vi "Read Data.vi"(8 "error in (no error)":errorcluster, 11 "LakeShore 335 in":refnum<class "LakeShore 335.lvclass">) -> (0 "error out":errorcluster, 2 "Data":waveform(dbl)[](array[waveform]), 3 "LakeShore 335 out":refnum<class "LakeShore 335.lvclass">)   [LabVIEW 2015, in "LakeShore 335.lvclass"]
uses:
  LakeShore 335.lvclass
  LakeShore335 Front Panel Data.ctl
  LakeShore335 Heater Ranges.ctl
  Neocera/Neocera Set Point Aproach.ctl
  OO Devices/Device/Read Controls Snapshot.vi
  Instrument/Read VISA Resource.vi
  OO Devices/Device/Read Control Panel Loaded.vi
  Instrument/Write VISA Resource.vi
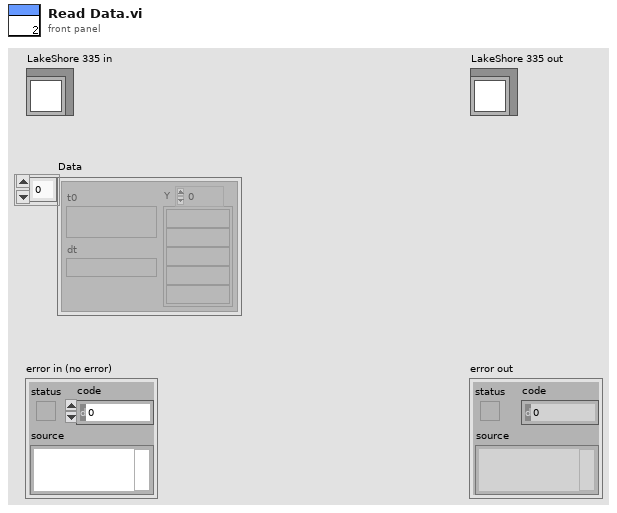
[diagram p1: front panel]
types:
  T1 = typedef "LakeShore335 Front Panel Data.ctl" = cluster{"Heater":bool, "A":bool, "B":bool, " RAW":bool, "Set point":dbl, "Set Heater Range":T2, "Approach":T3, "Ramp rate, K/min":dbl}
  T2 = typedef "LakeShore335 Heater Ranges.ctl" = enum16{"0 (Off)", "1 Low", "2 Medium", "3 High"}
  T3 = typedef "Neocera Set Point Aproach.ctl" = enum16{"Instant", "Ramp"}
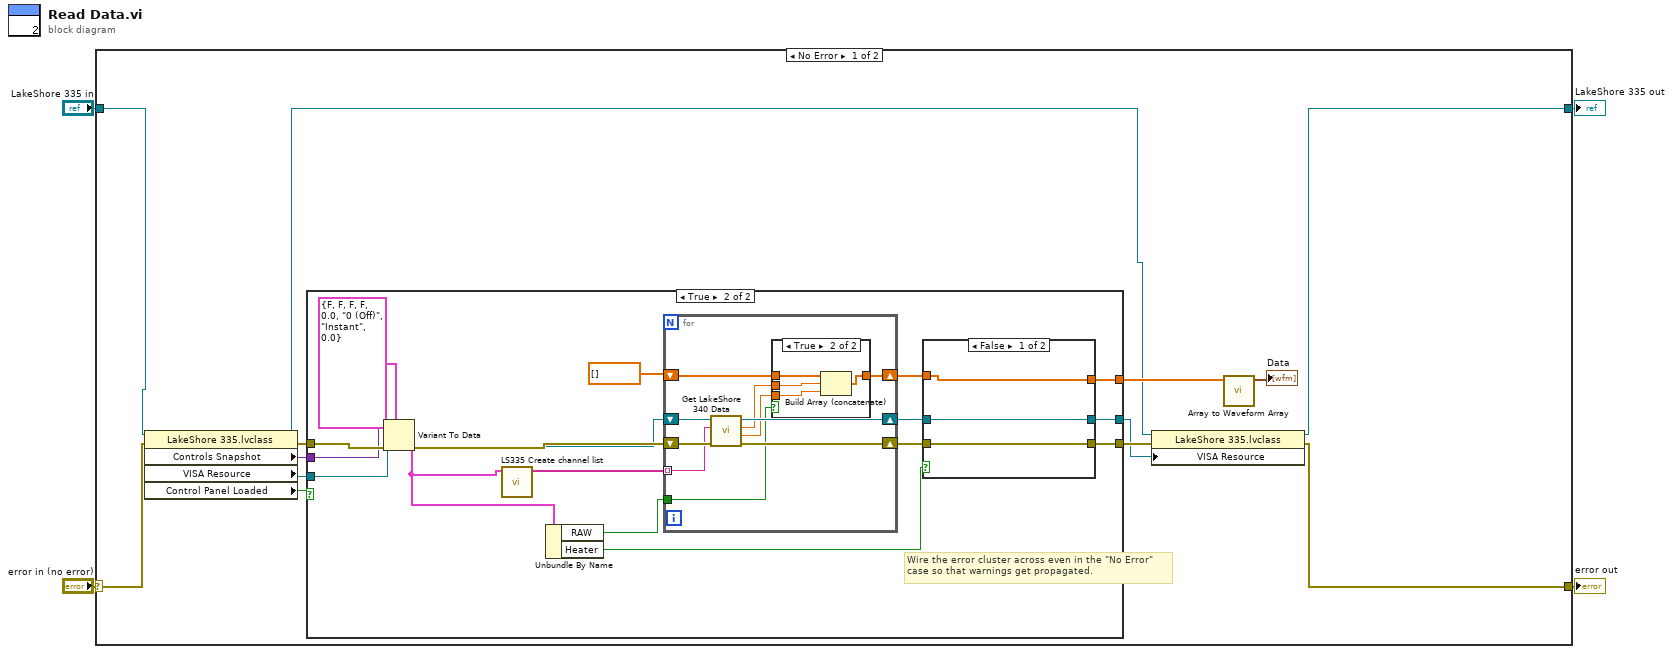
[diagram p0: block diagram]
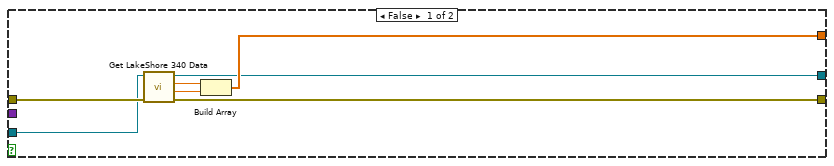
[diagram p2: hidden frame]
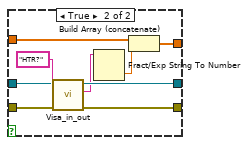
[diagram p3: hidden frame]
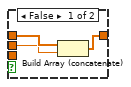
[diagram p4: hidden frame]
diagram:
  n1 = case shown="No Error" "error in (no error)" {
    selector: "error in (no error)" -> [w9 w71]
    tunnel: [w5 w71] -> w3
    tunnel: [w6 w70] -> w1
    tunnel: "LakeShore 335 in" -> [w8 w70]
    frame No Error {
      # "Wire the error cluster across even in the \"No Error\"\ncase so that warnings get propagated."
      n2 = property class="LakeShore 335.lvclass"(reference=w8, error in=w9) -> (reference out=w7:refnum<class "LakeShore 335.lvclass">, error out=w16:errorcluster, "Controls Snapshot"=w15:variant, "VISA Resource"=w12:refnum<visa-resource-name>, "Control Panel Loaded"=w11:bool)
      n3 = case shown="True" w11 {
        tunnel: w16 -> [w24 w40]
        tunnel: w15 -> [_ w39]
        tunnel: [w22 w33] -> w14
        tunnel: [w19 w30] -> w13
        tunnel: w12 -> [w23 w28]
        tunnel: [w18 w27] -> w10
        frame False {
          n4 = call "Get LakeShore 340 Data.vi"("error in (no error)"=w24, "VISA Resource Name"=w23) -> ("error out"=w22:errorcluster, "Raw"=w20:dbl, "Temperature"=w21:dbl, "VISA Resource Name Out"=w18:refnum<visa-resource-name>)  [unwired: 1 in, 5 out]
          n5 = Build Array(w21, w20) -> (w19:dbl[])
        }
        frame True {
          n6 = Variant To Data(error in=w40, type=T1 {"Heater"=FALSE, "A"=FALSE, "B"=FALSE, " RAW"=FALSE, "Set point"=0.0, "Set Heater Range"=enum."0 (Off)", "Approach"=enum."Instant", "Ramp rate, K/min"=0.0} ("Data"), Variant=w39) -> (data=w26:T1, error out=w29:errorcluster)
          n7 = call "LS335 Create channel list.vi"("Data"=w26) -> ("Array"=w25:string[])  [unwired: 10 in]
          n8 = Unbundle By Name(w26) -> ("RAW"=w36:bool, "Heater"=w35:bool)
          n9 = for {
            shift-right: [w62] -> w34
            shift-left: w29 -> [w61]
            shift-right: [w60] -> w32
            shift-left: w28 -> [w59]
            shift-right: [w56] -> w31
            shift-left: dbl[] [] -> [w58]
            tunnel: w36 -> [w54]
            tunnel: w25 -> [w53] mode=indexing
            n10 = call "Get LakeShore 340 Data.vi"("error in (no error)"=w61, "Input (A or B)"=w53, "VISA Resource Name"=w59) -> ("error out"=w62:errorcluster, "Raw"=w55:dbl, "Temperature"=w57:dbl, "VISA Resource Name Out"=w60:refnum<visa-resource-name>)  [unwired: 5 out]
            n11 = case shown="True" w54 {
              tunnel: w58 -> [w65 w69]
              tunnel: w57 -> [w63 w68]
              tunnel: [w64 w67] -> w56
              tunnel: w55 -> [_ w66]
              frame False {
                n12 = Build Array (concatenate)(w65, w63) -> (w64:dbl[])
              }
              frame True {
                n13 = Build Array (concatenate)(w69, w68, w66) -> (w67:dbl[])
              }
            }
          }
          n14 = case shown="False" w35 {
            tunnel: w34 -> [w43 w51]
            tunnel: [w43 w50] -> w33
            tunnel: [w42 w49] -> w27
            tunnel: w32 -> [w42 w48]
            tunnel: w31 -> [w41 w46]
            tunnel: [w41 w44] -> w30
            frame False {
            }
            frame True {
              n15 = call "Visa_in_out.vi"("error in (no error)"=w51, "write buffer"="HTR?", "VISA resource name"=w48) -> ("error out"=w50:errorcluster, "read buffer"=w47:string, "VISA resource name out"=w49:refnum<visa-resource-name>)  [unwired: 1 in, 5 out]
              n16 = Fract/Exp String To Number(string=w47) -> (number=w45:dbl)  [unwired: 1 in, 3 out]
              n17 = Build Array (concatenate)(w46, w45) -> (w44:dbl[])
            }
          }
        }
      }
      n18 = property class="LakeShore 335.lvclass"(reference=w7, error in=w14, "VISA Resource"=w10) -> (reference out=w6:refnum<class "LakeShore 335.lvclass">, error out=w5:errorcluster)
      n19 = call "Array to Waveform Array.vi"("Array"=w13) -> ("Waveform"=→"Data":waveform(dbl)[])  [unwired: 10 in]
    }
    frame Error {
    }
  }
  "error out" <- w3
  "LakeShore 335 out" <- w1
